vi "Math-N Point Smooth.vi"(0 "Array":dbl[](array[numeric]), 7 "Span (3)":i32=3) -> (4 "Smoothed Array":dbl[](array[numeric]))   [LabVIEW 2015]
uses:
  <vilib>/Analysis/2dsp.llb/1D Convolution (DBL).vi
  <vilib>/Analysis/NI_AALPro.lvlib
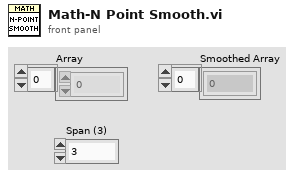
[diagram p1: front panel]
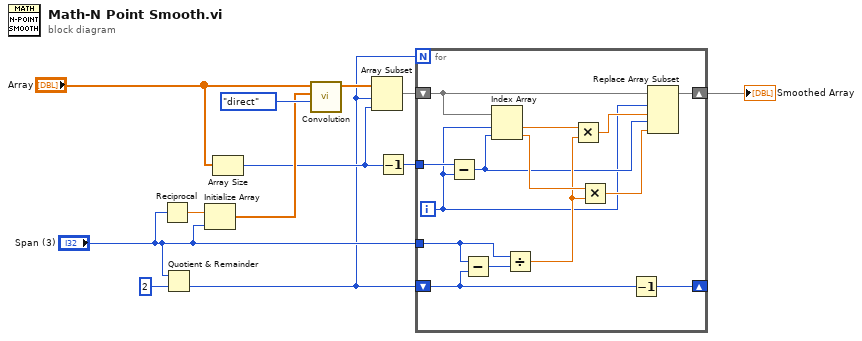
[diagram p0: block diagram]
diagram:
  n1 = Reciprocal(x="Span (3)") -> (1/x=w4:dbl)
  n2 = Quotient & Remainder(x="Span (3)", y=2) -> (floor(x/y)=w1:i32)  [unwired: 1 out]
  n3 = Initialize Array(w4, "Span (3)") -> (w5:dbl[])
  n4 = Array Size(array="Array") -> (size(s)=w3:i32)
  n5 = call-poly <vilib>:"Convolution.vi"("algorithm"=enum32{"direct", "frequency domain"}."direct", "Y"=w5, "X"="Array") -> ("X * Y"=w8:dbl[])  [unwired: 7 in, 1 out]
  n6 = Array Subset(array=w8, index=w1, length=w3) -> (w10:dbl[])
  n7 = Decrement(x=w3) -> (x-1=w2:i32)
  n8 = for {
    N: w1 -> [_]
    shift-right: [w25] -> w11
    shift-left: w10 -> [w26]
    tunnel: "Span (3)" -> [w22]
    tunnel: w2 -> [w20]
    shift-right: [w13] -> _
    shift-left: w1 -> [w14]
    i -> [w15]
    n9 = Subtract(x=w20, y=w15) -> (x-y=w17:i32)
    n10 = Subtract(x=w22, y=w14) -> (x-y=w23:i32)
    n11 = Index Array(array=w26, index #1=w15, index #2=w17) -> (element #1=w24:dbl, element #2=w19:dbl)
    n12 = Divide(x=w22, y=w23) -> (x/y=w18:dbl)
    n13 = Multiply(x=w24, y=w18) -> (x*y=w21:dbl)
    n14 = Multiply(x=w19, y=w18) -> (x*y=w16:dbl)
    n15 = Decrement(x=w14) -> (x-1=w13:i32)
    n16 = Replace Array Subset(array=w26, new element #1=w21, index #1=w15, new element #2=w16, index #2=w17) -> (w25:dbl[])
  }
  "Smoothed Array" <- w11
